vi "parseCommand.vi"(8 "error in (no error)":errorcluster, 10 "command in":string, 11 "CoolerSerialCommand in":refnum<class "CoolerSerialCommand.lvclass">) -> (0 "error out":errorcluster, 2 "command out":T1, 3 "CoolerSerialCommand out":refnum<class "CoolerSerialCommand.lvclass">)   [LabVIEW 2016, in "CoolerSerialCommand.lvclass"]
uses:
  CoolerSerialCommand.lvclass
  typedefs/command.ctl
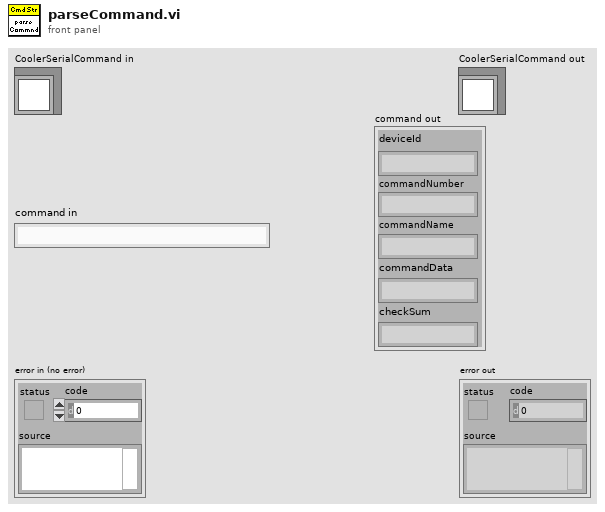
[diagram p1: front panel]
types:
  T1 = typedef "command.ctl" = cluster{"deviceId":string, "commandNumber":string, "commandName":string, "commandData":string, "checkSum":string}
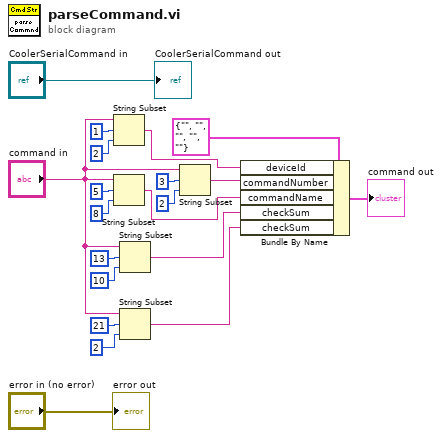
[diagram p0: block diagram]
diagram:
  n1 = String Subset(string="command in", offset (0)=1, length (rest)=2 ("offset (0)")) -> (substring=w17:string)
  n2 = String Subset(string="command in", offset (0)=5, length (rest)=8 ("offset (0)")) -> (substring=w14:string)
  n3 = String Subset(string="command in", offset (0)=13, length (rest)=10 ("offset (0)")) -> (substring=w15:string)
  n4 = String Subset(string="command in", offset (0)=21, length (rest)=2 ("offset (0)")) -> (substring=w18:string)
  n5 = String Subset(string="command in", offset (0)=3, length (rest)=2 ("offset (0)")) -> (substring=w16:string)
  n6 = Bundle By Name(cluster=T1 {"deviceId"="", "commandNumber"="", "commandName"="", "commandData"="", "checkSum"=""} ("command"), "deviceId"=w17, "commandNumber"=w16, "commandName"=w14, "checkSum"=w15, "checkSum"=w18) -> (→"command out":T1)
  "error out" <- "error in (no error)"
  "CoolerSerialCommand out" <- "CoolerSerialCommand in"
